vi "ArmAtSetpoint.vi"(8 "ArmSetpoints":T1) -> (0 "AtSetpoint":bool)   [LabVIEW 2023]
doc: "Makes sure the actual position of the arm is within 5 degrees of the setpoint/target"
uses:
  ArmGetSetpointEnum.ctl
  ArmGlobal.vi
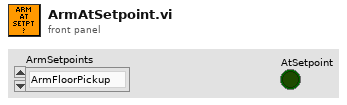
[diagram p1: front panel]
types:
  T1 = typedef "ArmGetSetpointEnum.ctl" = enum16{"ArmFloorPickup", "ArmAmpDeposit", "ArmSpeakerShoot", "ArmStartPosition", "ArmRestPosition", "ArmSourceIntake", "ArmAwayShoot"}
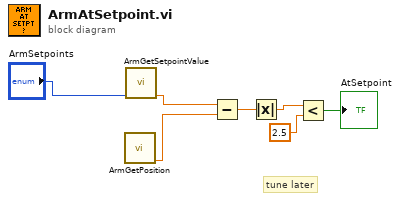
[diagram p0: block diagram]
diagram:
  # "tune later"
  n1 = call "ArmGetPosition.vi"() -> ("ArmPos"=w5:dbl)  [unwired: 11 in]
  n2 = call "ArmGetSetpointValue.vi"("ArmSetpoints"="ArmSetpoints") -> ("Setpoint"=w6:dbl)  [unwired: 10 in]
  n3 = Subtract(x=w6, y=w5) -> (x-y=w4:dbl)
  n4 = Absolute Value(x=w4) -> (abs(x)=w3:dbl)
  n5 = Less?(x=w3, y=2.5) -> (x < y?=→"AtSetpoint":bool)
